vi "guards.vi"(6 "state data":T4={"auto play?"=FALSE, "good disc?"=FALSE, "last action"=enum."start_playback", "track #"=0, "# tracks"=0, "repeat"=enum."none"}, 9 "event":T2, 10 "state":T3, 11 "guard":T1) -> (0 "error out":errorcluster, 3 "pass guard?":bool)   [LabVIEW 2019, in "test-state-machine.lvlib"]
uses:
  test-state-machine.lvlib
  State Data.ctl
  Action Type.ctl
  State Type.ctl
  Event Type.ctl
  Guard Type.ctl
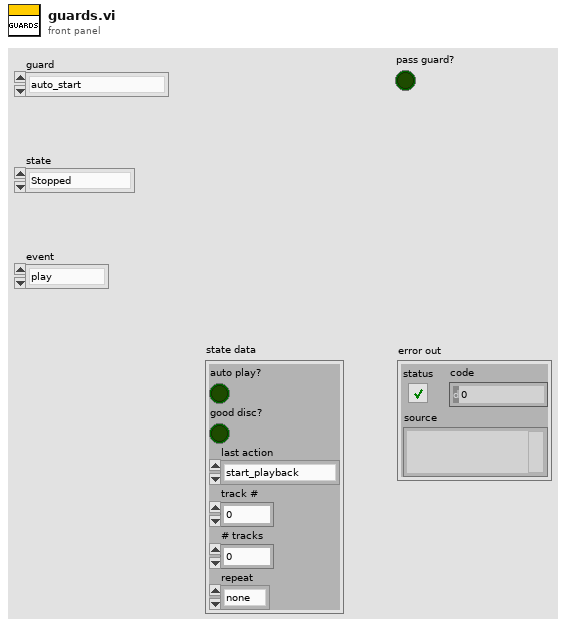
[diagram p1: front panel]
types:
  T1 = typedef "test-state-machine.lvlib/Guard Type.ctl" = enum16{"auto_start", "good_disk_format", "has_next_track", "has_prev_track", "repeat_one", "last_track_and_repeat", "last_track"}
  T2 = typedef "test-state-machine.lvlib/Event Type.ctl" = enum16{"play", "open_close", "stop", "cd_detected", "pause", "end_pause", "track_done", "autoplay", "error", "repeat_mode", "next", "previous"}
  T3 = typedef "test-state-machine.lvlib/State Type.ctl" = enum16{"Stopped", "Open", "Empty", "Playing", "Paused", "Error"}
  T4 = typedef "test-state-machine.lvlib/State Data.ctl" = cluster{"auto play?":bool, "good disc?":bool, "last action":T5, "track #":u8, "# tracks":u8, "repeat":enum16{"none", "one", "all"}}
  T5 = typedef "test-state-machine.lvlib/Action Type.ctl" = enum16{"null action", "start_playback", "open_drawer", "close_drawer", "store_cd_info", "stop_playback", "pause_playback", "stop_and_open", "resume_playback", "next_track", "prev_track", "repeat_track", "play_first", "toggle_autoplay", "stop_safe", "toggle_repeat_mode"}
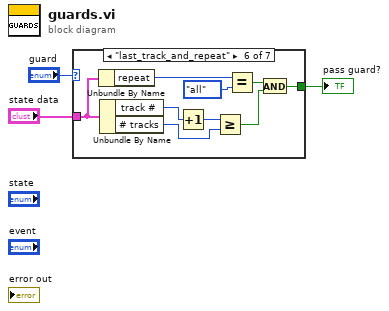
[diagram p0: block diagram]
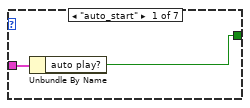
[diagram p2: hidden frame]
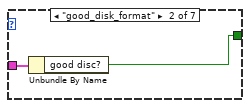
[diagram p3: hidden frame]
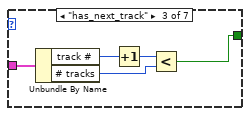
[diagram p4: hidden frame]
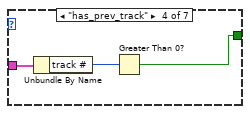
[diagram p5: hidden frame]
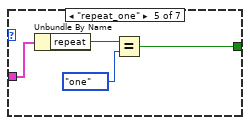
[diagram p6: hidden frame]
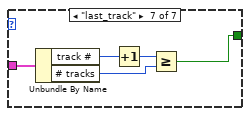
[diagram p7: hidden frame]
diagram:
  n1 = case shown="\"last_track_and_repeat\"" "guard" {
    tunnel: [w4 w6 w9 w14 w16 w20 w32] -> w2
    tunnel: "state data" -> [w5 w7 w12 w15 w17 w23 w33]
    frame "auto_start" {
      n2 = Unbundle By Name(w5) -> ("auto play?"=w4:bool)
    }
    frame "good_disk_format" {
      n3 = Unbundle By Name(w7) -> ("good disc?"=w6:bool)
    }
    frame "has_next_track" {
      n4 = Unbundle By Name(w12) -> ("track #"=w11:u8, "# tracks"=w10:u8)
      n5 = Increment(x=w11) -> (x+1=w8:u8)
      n6 = Less?(x=w8, y=w10) -> (x < y?=w9:bool)
    }
    frame "has_prev_track" {
      n7 = Unbundle By Name(w15) -> ("track #"=w13:u8)
      n8 = Greater Than 0?(x=w13) -> (x > 0?=w14:bool)
    }
    frame "repeat_one" {
      n9 = Unbundle By Name(w17) -> ("repeat"=w19:enum16{"none", "one", "all"})
      n10 = Equal?(x=w19, y=enum16{"none", "one", "all"}."one") -> (x = y?=w16:bool)
    }
    frame "last_track_and_repeat" {
      n11 = Unbundle By Name(w23) -> ("repeat"=w28:enum16{"none", "one", "all"})
      n12 = Unbundle By Name(w23) -> ("track #"=w26:u8, "# tracks"=w25:u8)
      n13 = Increment(x=w26) -> (x+1=w24:u8)
      n14 = Greater Or Equal?(x=w24, y=w25) -> (x >= y?=w21:bool)
      n15 = Equal?(x=w28, y=enum16{"none", "one", "all"}."all") -> (x = y?=w22:bool)
      n16 = And(x=w22, y=w21) -> (x .and. y?=w20:bool)
    }
    frame "last_track" {
      n17 = Unbundle By Name(w33) -> ("track #"=w31:u8, "# tracks"=w30:u8)
      n18 = Increment(x=w31) -> (x+1=w29:u8)
      n19 = Greater Or Equal?(x=w29, y=w30) -> (x >= y?=w32:bool)
    }
  }
  "pass guard?" <- w2
